vi "Change All Channel Tags.vi"(8 "error in (no error)":errorcluster, 10 "Name":string, 11 "Section Ref in":T1 format="%.0x") -> (0 "error out":errorcluster)   [LabVIEW 2013, in "OPC UA Client System Explorer.lvlib"]
uses:
  OPC UA Client System Explorer.lvlib
  <vilib>/NI Veristand/Custom Device API/Custom Device Item Ref.ctl
  Shared/Constants.vi
  <vilib>/NI Veristand/Custom Device Tools/Custom Device Utility Library/NI VeriStand - Search for All Items by GUID.vi
  <vilib>/NI Veristand/Custom Device API/Get Item Property (String).vi
  <vilib>/NI Veristand/Custom Device API/Set Item Property (String).vi
  <vilib>/NI Veristand/Custom Device Tools/Custom Device Utility Library/Custom Device Utility Library.lvlib
  Shared/OPC UA Client Shared.lvlib
  <vilib>/NI Veristand/Custom Device API/Custom Device API.lvlib
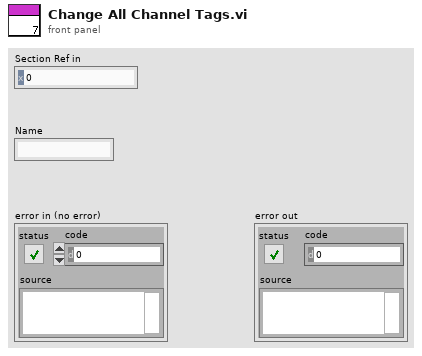
[diagram p1: front panel]
types:
  T1 = typedef "Custom Device API.lvlib/Custom Device Item Ref.ctl" = u64
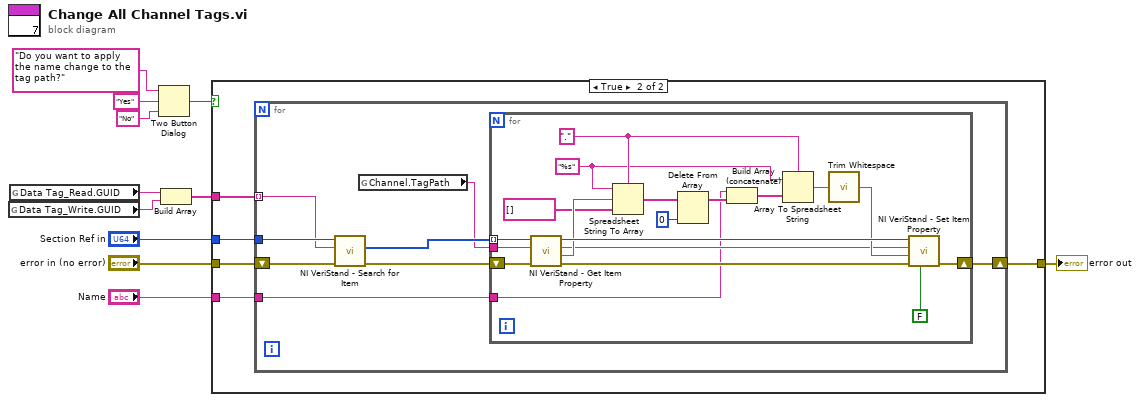
[diagram p0: block diagram]
diagram:
  n1 = global read "Constants.vi" "Data Tag_Write.GUID"() -> (w3:string)
  n2 = global read "Constants.vi" "Data Tag_Read.GUID"() -> (w4:string)
  n3 = Two Button Dialog(message="Do you want to apply the name change to the tag path?", 1:"No" ("F button name (\"Cancel\")"), 2:"Yes" ("T button name (\"OK\")")) -> (T button?=w9:bool)
  n4 = Build Array(w4, w3) -> (w2:string[])
  n5 = case shown="True" w9 {
    tunnel: "error in (no error)" -> [w12 w17]
    tunnel: [w12 w16] -> w11
    tunnel: "Section Ref in" -> [_ w15]
    tunnel: w2 -> [_ w14]
    tunnel: "Name" -> [_ w13]
    frame False {
    }
    frame True {
      n6 = for {
        shift-right: [w20] -> w16
        shift-left: w17 -> [w25]
        tunnel: w15 -> [w24]
        tunnel: w14 -> [w23] mode=indexing
        tunnel: w13 -> [w18]
        n7 = call-poly <vilib>:"NI VeriStand - Search for Item.vi"("error in"=w25, "Item GUID"=w23, "Section Ref in"=w24) -> ("error out"=w21:errorcluster, "Item Refs"=w22:T1[])  [unwired: 5 in, 2 out]
        n8 = global read "Constants.vi" "Channel.TagPath"() -> (w19:string)
        n9 = for {
          tunnel: w22 -> [w43] mode=indexing
          shift-right: [w40] -> w20
          shift-left: w21 -> [w42]
          tunnel: w19 -> [w27]
          tunnel: w18 -> [w26]
          w35 = "%s" ("format string")
          w36 = "." ("delimiter (Tab)")
          n10 = call-poly <vilib>:"NI VeriStand - Get Item Property.vi"("error in (no error)"=w42, "Property Name"=w27, "Item Ref in"=w43) -> ("error out"=w41:errorcluster, "Value"=w37:string, "Item Ref out"=w38:T1)  [unwired: 5 in, 1 out]
          n11 = Spreadsheet String To Array(delimiter (Tab)=w36, format string=w35, spreadsheet string=w37, array type (2D Dbl)=string[] []) -> (array=w33:string[])
          n12 = Delete From Array(array=w33, index=0) -> (array with subset deleted=w31:string[])  [unwired: 1 in, 1 out]
          n13 = Build Array (concatenate)(w26, w31) -> (w30:string[])
          n14 = Array To Spreadsheet String(delimiter (Tab)=w36, array=w30, 3:w35) -> (spreadsheet string=w29:string)
          n15 = call <vilib>:"Trim Whitespace.vi"("string"=w29) -> ("trimmed string"=w28:string)  [unwired: 1 in]
          n16 = call-poly <vilib>:"NI VeriStand - Set Item Property.vi"("Binary String (T)"=FALSE, "error in (no error)"=w41, "Value"=w28, "Property Name"=w27, "Item Ref in"=w38) -> ("error out"=w40:errorcluster)  [unwired: 4 in, 2 out]
        }
      }
    }
  }
  "error out" <- w11
